vi "P.AverageSubVi.vi"(1 "Array":dbl[][](array[numeric])) -> (0 "output array":dbl[][][](array[numeric]))   [LabVIEW 2021]
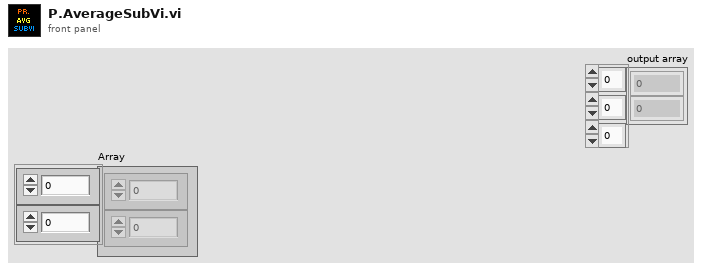
[diagram p1: front panel]
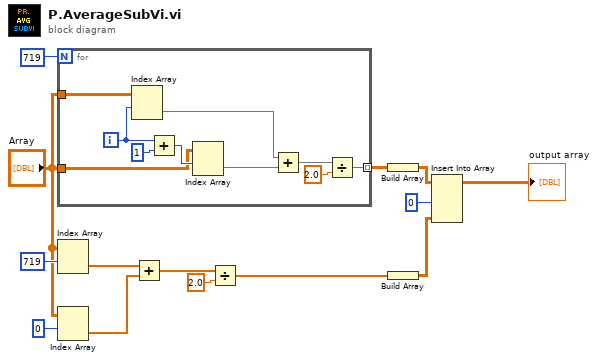
[diagram p0: block diagram]
diagram:
  n1 = for {
    N: 719 -> [_]
    tunnel: "Array" -> [w24]
    tunnel: "Array" -> [w19]
    tunnel: [w15] -> w4 mode=indexing
    i -> [w22]
    n2 = Index Array "Index Array"(array=w24, index (row)=w22) -> (element=w20:dbl[])  [unwired: 1 in]
    n3 = Add(x=w22, y=1) -> (x+y=w21:i32)
    n4 = Index Array "Index Array"(array=w19, index (row)=w21) -> (element=w18:dbl[])  [unwired: 1 in]
    n5 = Add(x=w20, y=w18) -> (x+y=w17:dbl[])
    n6 = Divide(x=w17, y=2.0) -> (x/y=w15:dbl[])
  }
  n7 = Index Array "Index Array"(array="Array", index (row)=719 ("index")) -> (element=w12:dbl[])  [unwired: 1 in]
  n8 = Index Array "Index Array"(array="Array", index (row)=0 ("index")) -> (element=w11:dbl[])  [unwired: 1 in]
  n9 = Add(x=w12, y=w11) -> (x+y=w8:dbl[])
  n10 = Divide(x=w8, y=2.0) -> (x/y=w6:dbl[])
  n11 = Build Array(w4) -> (w3:dbl[][][])
  n12 = Build Array(w6) -> (w5:dbl[][])
  n13 = Insert Into Array "Insert Into Array"(array=w3, index (dim 1)=0 ("disabled index (row)"), new element=w5) -> (→"output array":dbl[][][])  [unwired: 2 in]
